vi "SetDriveTank.vi"(8 "error in":errorcluster, 10 "Right":dbl, 11 "Left":dbl) -> (0 "error out":errorcluster)   [LabVIEW 2016]
uses:
  Robot Global Data.vi
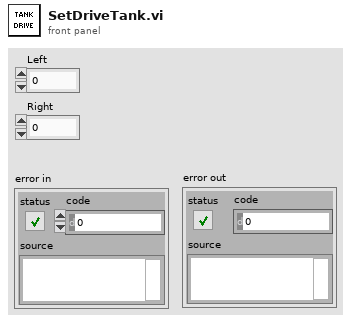
[diagram p1: front panel]
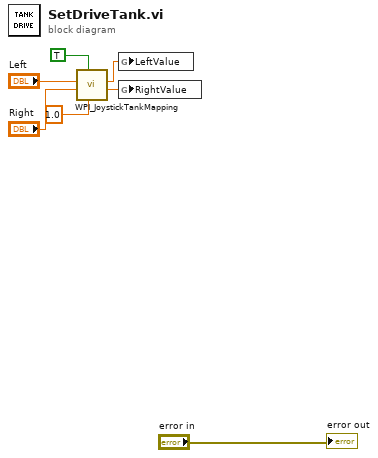
[diagram p0: block diagram]
diagram:
  n1 = call <vilib>:"WPI_JoystickTankMapping.vi"("Max Output"=1.0, "Square Inputs"=TRUE, "Right axis value"="Right", "Left axis value"="Left") -> ("Right Motor Value"=w2:dbl, "Left Motor Value"=w3:dbl)  [unwired: 6 in]
  n2 = global write "Robot Global Data.vi" "LeftValue"(w3) -> ()
  n3 = global write "Robot Global Data.vi" "RightValue"(w2) -> ()
  "error out" <- "error in"
